vi "CLI.vi"(11 "Command line arguments":string[](array[string])) -> (2 "Output/Error message":string, 3 "Return code":i32)   [LabVIEW 2019]
uses:
  Typedefs/Generation options.ctl
  Typedefs/Tab.ctl
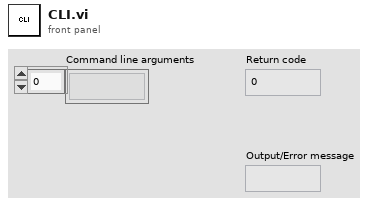
[diagram p1: front panel]
types:
  T1 = typedef "Generation options.ctl" = cluster{"Minify?":bool, "Disabled Tabs":T2[], "Default Tab":T2}
  T2 = typedef "Tab.ctl" = enum16{"Info", "FP", "BD"}
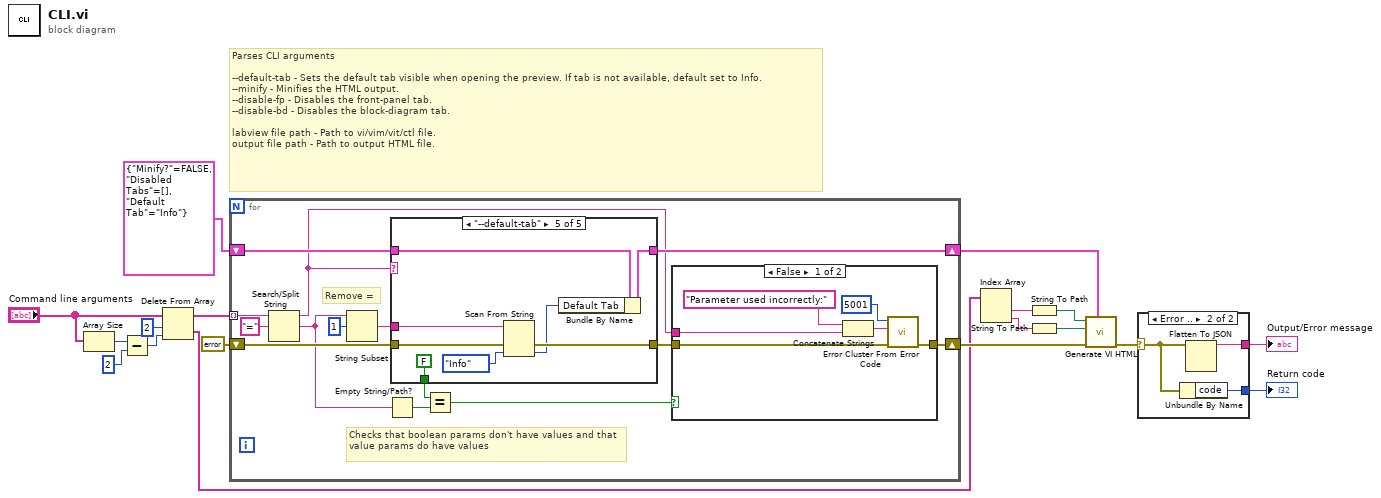
[diagram p0: block diagram]
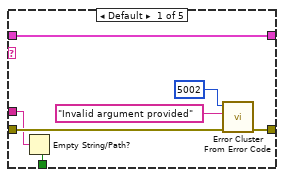
[diagram p3: hidden frame]
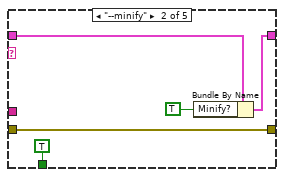
[diagram p4: hidden frame]
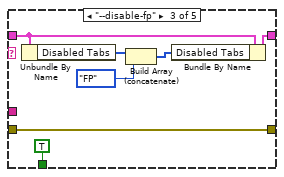
[diagram p5: hidden frame]
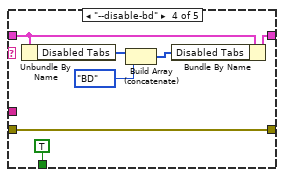
[diagram p6: hidden frame]
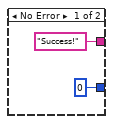
[diagram p7: hidden frame]
diagram:
  # "Parses CLI arguments\n\n--default-tab - Sets the default tab visible when opening the preview. If tab is not available, default set to Info.\n--minify - Minifies the HTML output.\n--disable-fp - Disables the front-panel tab.\n--disable-bd - Disables the block-diagram tab.\n\nlabview file path - Path to vi/vim/vit/ctl file.\noutput file path - Path to output HTML file."
  n1 = Array Size(array="Command line arguments") -> (size(s)=w13:i32)
  n2 = Subtract(x=w13, y=2) -> (x-y=w11:i32)
  n3 = Delete From Array(array="Command line arguments", length=2, index=w11) -> (deleted portion=w6:string[], array with subset deleted=w15:string[])
  n4 = for {
    shift-right: [w29] -> w9
    shift-left: T1 {"Minify?"=FALSE, "Disabled Tabs"=[], "Default Tab"=enum."Info"} ("Generation options") -> [w30]
    tunnel: w15 -> [w32] mode=indexing
    shift-right: [w24] -> w8
    shift-left: errorcluster {"status"=FALSE, "code"=0, "source"=""} ("error IO") -> [w26]
    # "Remove ="
    # "Checks that boolean params don't have values and that value params do have values"
    n5 = Search/Split String(string=w32, search string/char (-)="=") -> (substring before match=w22:string, match + rest of string=w20:string)  [unwired: 1 in, 1 out]
    n6 = String Subset(string=w20, offset (0)=1) -> (substring=w19:string)  [unwired: 1 in]
    n7 = Empty String/Path?(string/path=w20) -> (empty?=w28:bool)
    n8 = case shown="\"--default-tab\"" w22 {
      tunnel: w30 -> [w40 w51 w55 w62 w68]
      tunnel: [w40 w50 w58 w65 w67] -> w29
      tunnel: w19 -> [w42 _ _ _ w71]
      tunnel: [w41 TRUE TRUE TRUE FALSE] -> w27
      tunnel: [w45 w47 w56 w63 w72] -> w25
      tunnel: w26 -> [w46 w47 w56 w63 w73]
      frame Default {
        n9 = Empty String/Path?(string/path=w42) -> (empty?=w41:bool)
        n10 = call <vilib>:"Error Cluster From Error Code.vi"("error in (no error)"=w46, "error message (\"\")"="Invalid argument provided" ("error message (\"\")"), "error code (0)"=5002) -> ("error out"=w45:errorcluster)  [unwired: 6 in]
      }
      frame "--minify" {
        n11 = Bundle By Name(cluster=w51, "Minify?"=TRUE) -> (w50:T1)
      }
      frame "--disable-fp" {
        n12 = Unbundle By Name(w55) -> ("Disabled Tabs"=w54:T2[])
        n13 = Build Array (concatenate)(w54, Tab."FP" ("array")) -> (w53:T2[])
        n14 = Bundle By Name(cluster=w55, "Disabled Tabs"=w53) -> (w58:T1)
      }
      frame "--disable-bd" {
        n15 = Unbundle By Name(w62) -> ("Disabled Tabs"=w61:T2[])
        n16 = Build Array (concatenate)(w61, Tab."BD" ("array")) -> (w60:T2[])
        n17 = Bundle By Name(cluster=w62, "Disabled Tabs"=w60) -> (w65:T1)
      }
      frame "--default-tab" {
        n18 = Scan From String(input string=w71, error in=w73, default 1=Tab."Info" ("Default Tab")) -> (error out=w72:errorcluster, output 1=w66:T2)  [unwired: 2 in, 2 out]
        n19 = Bundle By Name(cluster=w68, "Default Tab"=w66) -> (w67:T1)
      }
    }
    n20 = Equal?(x=w27, y=w28) -> (x = y?=w23:bool)
    n21 = case shown="False" w23 {
      tunnel: w25 -> [w37 w39]
      tunnel: [w36 w39] -> w24
      tunnel: w22 -> [w33 _]
      frame False {
        n22 = Concatenate Strings("Parameter used incorrectly:" ("error message (\"\")"), w33) -> (w34:string)
        n23 = call <vilib>:"Error Cluster From Error Code.vi"("error in (no error)"=w37, "error message (\"\")"=w34, "error code (0)"=5001) -> ("error out"=w36:errorcluster)  [unwired: 6 in]
      }
      frame True {
      }
    }
  }
  n24 = Index Array(array=w6) -> (element #1=w4:string, element #2=w3:string)  [unwired: 2 in]
  n25 = String To Path(string=w4) -> (path=w18:path)
  n26 = String To Path(string=w3) -> (path=w5:path)
  n27 = call "Generate VI HTML.vi"("Generation options"=w9, "error in"=w8, "Output path"=w5, "VI Path"=w18) -> ("error out"=w2:errorcluster)  [unwired: 7 in]
  n28 = case shown="Error .." w2 {
    selector: w2 -> [_ w76]
    tunnel: [0 ("code") w77] -> w17
    tunnel: ["Success!" ("source") w78] -> w16
    frame No Error {
    }
    frame Error {
      n29 = Unbundle By Name(w76) -> ("code"=w77:i32)
      n30 = Flatten To JSON(anything=w76) -> (JSON string=w78:string)  [unwired: 2 in, 1 out]
    }
  }
  "Return code" <- w17
  "Output/Error message" <- w16
